vi "Read Y Scale.vi"(9 "GraphChart in":refnum<class "GraphChart.lvclass">) -> (3 "GraphChart out":refnum<class "GraphChart.lvclass">, 4 "Y scale":refnum<class "GraphScale.lvclass">)   [LabVIEW 2014, in "GraphChart.lvclass"]
uses:
  GraphChart.lvclass
  GraphScale/GraphScale.lvclass
  GraphChart.lvclass/GraphChart.ctl
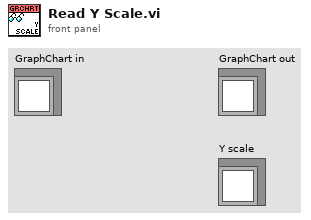
[diagram p1: front panel]
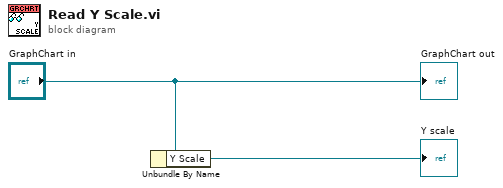
[diagram p0: block diagram]
diagram:
  n1 = Unbundle By Name("GraphChart in") -> ("Y Scale"=→"Y scale":refnum<class "GraphScale.lvclass">)
  "GraphChart out" <- "GraphChart in"
